vi "Replace Or Add Balls.vi"(10 "balls new":T1[](array[typedef]), 11 "balls":T1[](array[typedef])) -> (3 "Balls out":T1[](array[typedef]))   [LabVIEW 2016]
uses:
  SSL Detection Ball.ctl
  <vilib>/Analysis/Matrix/Datatypes/RealMatrix.ctl
  <vilib>/Analysis/Matrix/NI_Matrix.lvlib
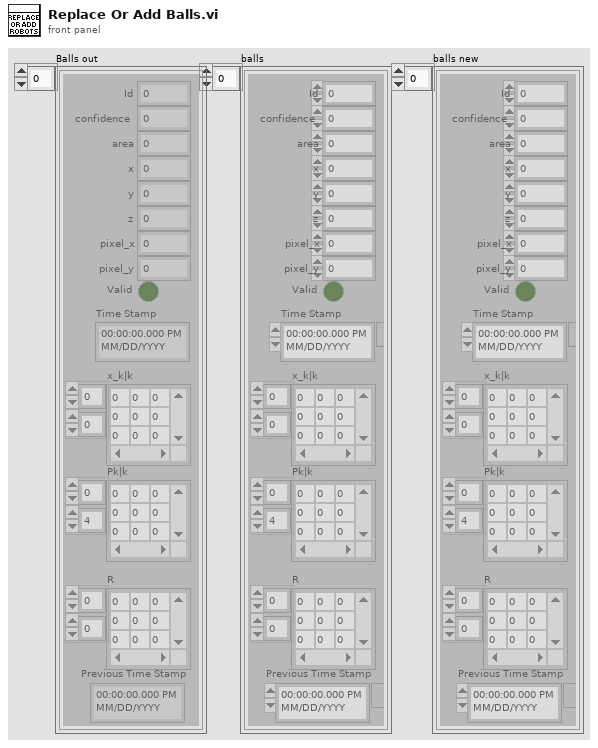
[diagram p1: front panel]
types:
  T1 = typedef "SSL Detection Ball.ctl" = cluster{"x":sgl, "area":u32, "confidence":sgl, "y":sgl, "z":sgl, "pixel_x":sgl, "pixel_y":sgl, "Valid":bool, "Time Stamp":timestamp, "x_k|k":T2, "Pk|k":T2, "Id":u32, "Previous Time Stamp":timestamp, "R":T2}
  T2 = typedef "NI_Matrix.lvlib/RealMatrix.ctl" = dbl[][]
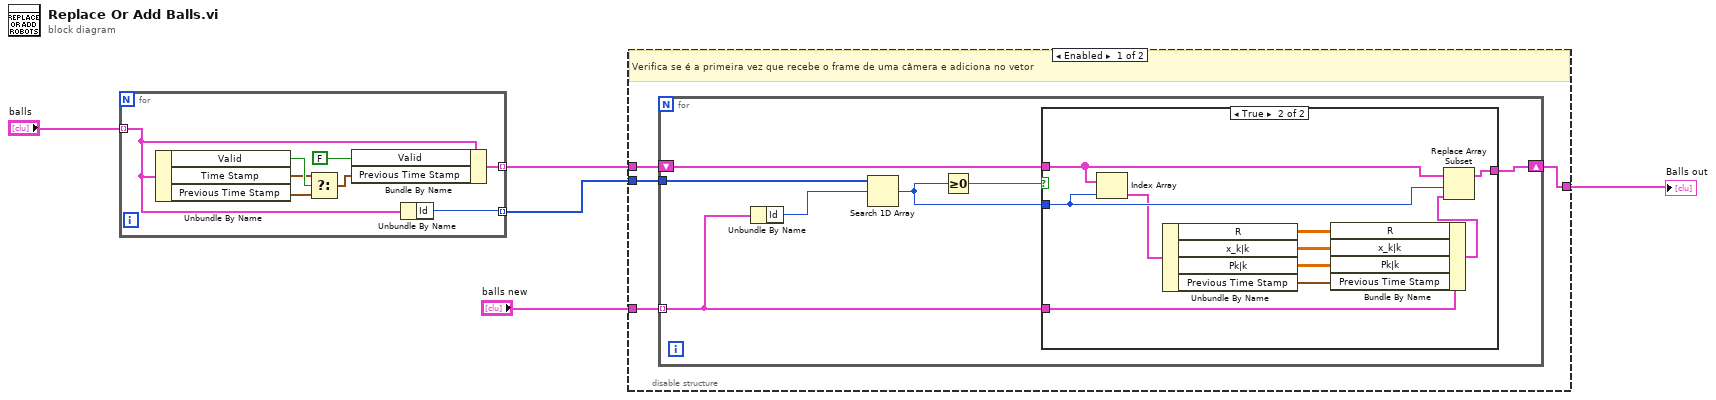
[diagram p0: block diagram]
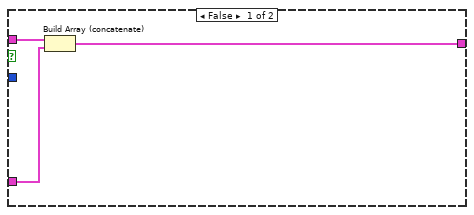
[diagram p2: hidden frame]
diagram:
  n1 = for {
    tunnel: "balls" -> [w10] mode=indexing
    tunnel: [w13] -> w5 mode=indexing
    tunnel: [w11] -> w4 mode=indexing
    n2 = Unbundle By Name(w10) -> ("Valid"=w9:bool, "Time Stamp"=w8:timestamp, "Previous Time Stamp"=w6:timestamp)
    n3 = Select(t=w8, s=w9, f=w6) -> (s? t:f=w7:timestamp)
    n4 = Bundle By Name(cluster=w10, "Valid"=FALSE, "Previous Time Stamp"=w7) -> (w11:T1)
    n5 = Unbundle By Name(w10) -> ("Id"=w13:u32)
  }
  n6 = disable-structure "Diagram Disable Structure" shown="Enabled" {
    disable-tunnel: w4 -> [w17 _]
    disable-tunnel: "balls new" -> [w16 _]
    disable-tunnel: [w15 _] -> w3
    disable-tunnel: w5 -> [w14 _]
    frame Enabled {
      # "Verifica se é a primeira vez que recebe o frame de uma câmera e adiciona no vetor"
      n7 = for {
        tunnel: w16 -> [w21] mode=indexing
        tunnel: w14 -> [w22]
        shift-right: [w23] -> w15
        shift-left: w17 -> [w24]
        n8 = Unbundle By Name(w21) -> ("Id"=w20:u32)
        n9 = Search 1D Array(1D array=w22, element=w20) -> (index of element=w18:i32)  [unwired: 1 in]
        n10 = Greater Or Equal To 0?(x=w18) -> (x >= 0?=w19:bool)
        n11 = case shown="True" w19 {
          tunnel: w24 -> [w27 w36]
          tunnel: w21 -> [w25 w33]
          tunnel: [w26 w37] -> w23
          tunnel: w18 -> [_ w35]
          frame False {
            n12 = Build Array (concatenate)(w27, w25) -> (w26:T1[])
          }
          frame True {
            n13 = Index Array(array=w36, index=w35) -> (element=w34:T1)
            n14 = Unbundle By Name(w34) -> ("R"=w28:T2, "x_k|k"=w31:T2, "Pk|k"=w30:T2, "Previous Time Stamp"=w29:timestamp)
            n15 = Bundle By Name(cluster=w33, "R"=w28, "x_k|k"=w31, "Pk|k"=w30, "Previous Time Stamp"=w29) -> (w32:T1)
            n16 = Replace Array Subset(array=w36, new element=w32, index=w35) -> (w37:T1[])
          }
        }
      }
    }
    frame Disabled {
    }
  }
  "Balls out" <- w3
